vi "Readout.vi"(8 "Error In":errorcluster, 11 "BNT_DAQmx-MCSV in":refnum<class "BNT_DAQmx-MCSV.lvclass">) -> (0 "Error Out":errorcluster, 2 "CSPP_DataCollection out":refnum<class "CSPP_DataCollection.lvclass">, 3 "BNT_DAQmx-MCSV out":refnum<class "BNT_DAQmx-MCSV.lvclass">)   [LabVIEW 2019, in "BNT_DAQmx.lvlib" / "BNT_DAQmx-MCSV.lvclass"]
doc: "Read single value from multiple channels."
uses:
  BNT_DAQmx-MCSV.lvclass
  CSPP_Core/Classes/CSPP_BaseClasses/DataCollection/CSPP_DataCollection.lvclass
  C:/User/Brand/LVP/LaserSpec/RADRIS/Packages/CSPP_Core/Actors/CSPP_BaseActor/CSPP_BaseActor.lvclass
  C:/Program Files (x86)/National Instruments/LabVIEW 2019/vi.lib/ActorFramework/Actor/Actor.lvclass
  CSPP_Core/Messages/CSPP_DataUpdate Msg/CSPP_DataUpdate Msg.lvclass
  BNT_DAQmx-MCSV-Data/BNT_DAQmx-MCSV-Data.lvclass
  C:/User/Brand/LVP/LaserSpec/RADRIS/Packages/CSPP_Core/Classes/CSPP_BaseClasses/Data/CSPP_Data.lvclass
  BNT_DAQmx-MCSV.lvclass/BNT_DAQmx-MCSV.ctl
  CSPP_Core/Actors/CSPP_BaseActor/CSPP_BaseActor.lvclass/CSPP_BaseActor.ctl
  CSPP_Core/Classes/CSPP_BaseClasses/Data/CSPP_Data.lvclass/CSPP_Data.ctl
  CSPP_Core/Classes/CSPP_BaseClasses/DataCollection/CSPP_DataCollection.lvclass/CSPP_DataCollection.ctl
  <vilib>/ActorFramework/Actor/Actor.lvclass/Actor.ctl
  <vilib>/ActorFramework/Message Enqueuer/Message Enqueuer.lvclass/Message Enqueuer.ctl
  <vilib>/DAQmx/read.llb/DAQmx Read (Counter 1D DBL NChan 1Samp).vi
  <vilib>/DAQmx/read.llb/DAQmx Read (Digital 1D Bool 1Chan 1Samp).vi
  CSPP_Core/Classes/CSPP_BaseClasses/Data/Write Error.vi
  CSPP_Core/Classes/CSPP_BaseClasses/Data/Write Time Stamp.vi
  <vilib>/ActorFramework/Message Enqueuer/Init from Existing Queue.vi
  <vilib>/DAQmx/miscellaneous.llb/DAQmx Fill In Error Info.vi
  <vilib>/ActorFramework/Message Enqueuer/Message Enqueuer.lvclass
  CSPP_Core/Actors/CSPP_BaseActor/CSPP_BaseActor.lvclass
  <vilib>/ActorFramework/Actor/Actor.lvclass
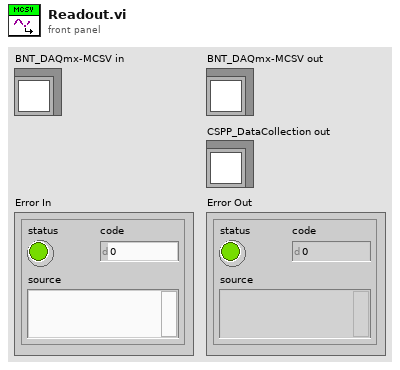
[diagram p1: front panel]
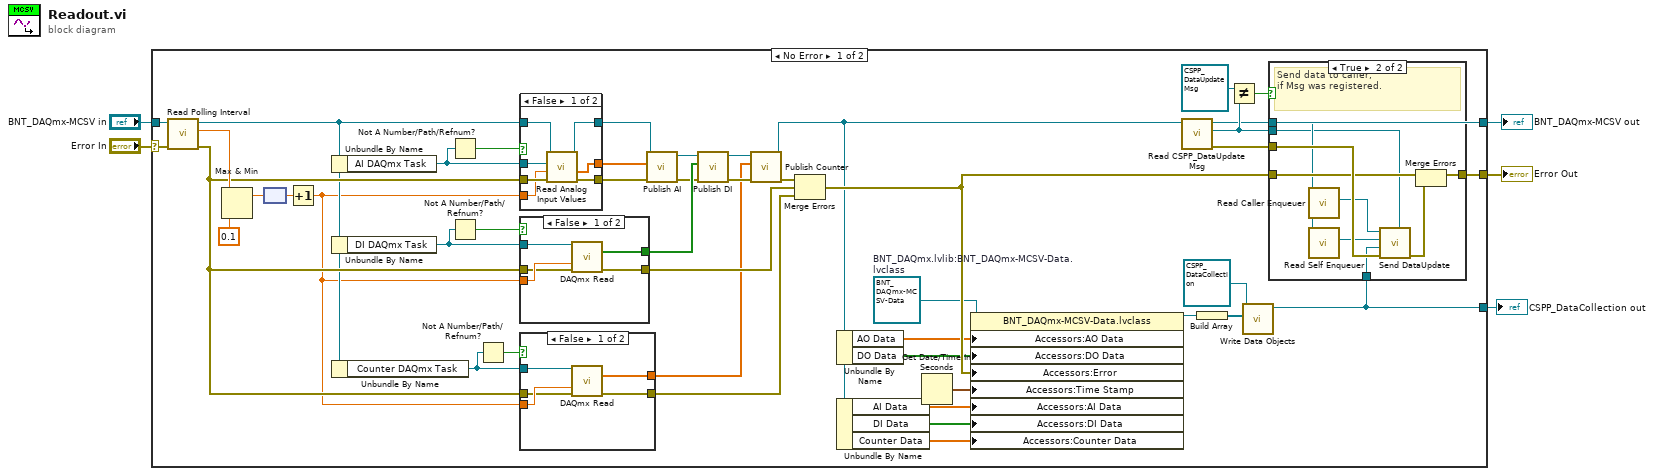
[diagram p0: block diagram]
diagram:
  n1 = case shown="No Error" "Error In" {
    selector: "Error In" -> [w50 w84]
    tunnel: [w38 w84] -> w4
    tunnel: [w20 w83] -> w2
    tunnel: "BNT_DAQmx-MCSV in" -> [w51 w83]
    tunnel: [w25 _] -> w1
    frame No Error {
      w32 = refnum<class "BNT_DAQmx-MCSV-Data.lvclass"> refnum  # BNT_DAQmx.lvlib:BNT_DAQmx-MCSV-Data.lvclass
      n2 = call "Read Polling Interval.vi"("error in (no error)"=w50, "CSPP_BaseActor in"=w51) -> ("error out"=w37:errorcluster, "Polling Interval"=w49:dbl[unit], "CSPP_BaseActor out"=w23:refnum<class "BNT_DAQmx-MCSV.lvclass">)  [unwired: 7 in]
      n3 = Max & Min(x=w49, y=dbl[unit] 0.1) -> (max(x,y)=w47:dbl[unit])  [unwired: 1 out]
      n4 = node(w47) -> (w40:dbl)
      n5 = Increment(x=w40) -> (x+1=w21:dbl)
      n6 = Unbundle By Name(w23) -> ("AI DAQmx Task"=w22:refnum<k21>)
      n7 = Unbundle By Name(w23) -> ("DI DAQmx Task"=w44:refnum<k21>)
      n8 = Unbundle By Name(w23) -> ("Counter DAQmx Task"=w41:refnum<k21>)
      n9 = Not A Number/Path/Refnum?(number/path/refnum=w22) -> (NaN/Path/Refnum?=w45:bool)
      n10 = Not A Number/Path/Refnum?(number/path/refnum=w44) -> (NaN/Path/Refnum?=w43:bool)
      n11 = Not A Number/Path/Refnum?(number/path/refnum=w41) -> (NaN/Path/Refnum?=w42:bool)
      n12 = case shown="False" w45 {
        tunnel: [w59 w66] -> w17
        tunnel: w21 -> [w62 _]
        tunnel: w37 -> [w63 w66]
        tunnel: w23 -> [w64 w65]
        tunnel: [w60 w65] -> w18
        tunnel: w22 -> [w61 _]
        tunnel: [w58 _] -> w16
        frame False {
          n13 = call-dynamic "Read Analog Input Values.vi"("error in"=w63, "Timeout / s"=w62, "AI DAQmx Task"=w61, "BNT_DAQmx-MCSV in"=w64) -> ("error out"=w59:errorcluster, "AI Data"=w58:dbl[], "BNT_DAQmx-MCSV out"=w60:refnum<class "BNT_DAQmx-MCSV.lvclass">)  [unwired: 5 in]
        }
        frame True {
        }
      }
      n14 = case shown="False" w43 {
        tunnel: w44 -> [w56 _]
        tunnel: w21 -> [w55 _]
        tunnel: [w52 _] -> w14
        tunnel: [w53 w57] -> w46
        tunnel: w37 -> [w54 w57]
        frame False {
          n15 = call-poly <vilib>:"DAQmx Read.vi"("task/channels in"=w56, "timeout"=w55, "error in"=w54) -> ("data"=w52:bool[], "error out"=w53:errorcluster)  [unwired: 10 in, 1 out]
        }
        frame True {
        }
      }
      n16 = case shown="False" w42 {
        tunnel: w41 -> [w71 _]
        tunnel: w21 -> [w70 _]
        tunnel: [w67 _] -> w8
        tunnel: [w68 w72] -> w39
        tunnel: w37 -> [w69 w72]
        frame False {
          n17 = call-poly <vilib>:"DAQmx Read.vi"("task/channels in"=w71, "timeout"=w70, "error in"=w69) -> ("data"=w67:dbl[], "error out"=w68:errorcluster)  [unwired: 10 in, 1 out]
        }
        frame True {
        }
      }
      n18 = call "Publish AI.vi"("error in"=w17, "AI Data"=w16, "BNT_DAQmx-MCSV in"=w18) -> ("error out"=w13:errorcluster, "BNT_DAQmx-MCSV out"=w12:refnum<class "BNT_DAQmx-MCSV.lvclass">)  [unwired: 7 in]
      n19 = call "Publish DI.vi"("error in"=w13, "DI Data"=w14, "BNT_DAQmx-MCSV in"=w12) -> ("error out"=w10:errorcluster, "BNT_DAQmx-MCSV out"=w11:refnum<class "BNT_DAQmx-MCSV.lvclass">)  [unwired: 7 in]
      n20 = call "Publish Counter.vi"("error in"=w10, "Counter Data"=w8, "BNT_DAQmx-MCSV in"=w11) -> ("error out"=w9:errorcluster, "BNT_DAQmx-MCSV out"=w6:refnum<class "BNT_DAQmx-MCSV.lvclass">)  [unwired: 7 in]
      n21 = Merge Errors(w9, w46, w39) -> (w35:errorcluster)
      n22 = Unbundle By Name(w6) -> ("AO Data"=w30:dbl[], "DO Data"=w29:bool[])
      n23 = Unbundle By Name(w6) -> ("AI Data"=w19:dbl[], "DI Data"=w15:bool[], "Counter Data"=w7:dbl[])
      n24 = Get Date/Time In Seconds() -> (seconds since 1Jan1904=w31:timestamp)
      n25 = property class="BNT_DAQmx-MCSV-Data.lvclass"(reference=w32, "Accessors:AO Data"=w30, "Accessors:DO Data"=w29, "Accessors:Error"=w35, "Accessors:Time Stamp"=w31, "Accessors:AI Data"=w19, "Accessors:DI Data"=w15, "Accessors:Counter Data"=w7) -> (reference out=w27:refnum<class "BNT_DAQmx-MCSV-Data.lvclass">)  [unwired: 1 in, 1 out]
      n26 = call-dynamic "Read CSPP_DataUpdate Msg.vi"("CSPP_BaseActor in"=w6) -> ("error out"=w36:errorcluster, "CSPP_DataUpdate Msg.lvclass"=w34:refnum<class "CSPP_DataUpdate Msg.lvclass">, "CSPP_BaseActor out"=w20:refnum<class "BNT_DAQmx-MCSV.lvclass">)  [unwired: 8 in]
      n27 = Build Array(w27) -> (w26:refnum<class "BNT_DAQmx-MCSV-Data.lvclass">[])
      n28 = Not Equal?(x=refnum<class "CSPP_DataUpdate Msg.lvclass"> refnum ("CSPP_DataUpdate Msg.lvclass"), y=w34) -> (x != y?=w24:bool)
      n29 = call "Write Data Objects.vi"("Data Objects"=w26, "CSPP_DataCollection in"=refnum<class "CSPP_DataCollection.lvclass"> refnum ("CSPP_BaseClasses.lvlib:CSPP_DataCollection.lvclass")) -> ("CSPP_DataCollection out"=w25:refnum<class "CSPP_DataCollection.lvclass">)  [unwired: 8 in, 1 out]
      n30 = case shown="True" w24 {
        tunnel: [w73 w82] -> w38
        tunnel: w36 -> [_ w81]
        tunnel: w35 -> [w73 w80]
        tunnel: w20 -> [_ w79]
        tunnel: w34 -> [_ w78]
        tunnel: w25 -> [_ w74]
        frame False {
        }
        frame True {
          # "Send data to caller, \nif Msg was registered."
          n31 = call <vilib>:"Read Caller Enqueuer.vi"("Actor"=w79) -> ("Caller Enqueuer"=w77:refnum<class "Message Enqueuer.lvclass">)  [unwired: 10 in]
          n32 = call <vilib>:"Read Self Enqueuer.vi"("Actor"=w79) -> ("Self Enqueuer"=w76:refnum<class "Message Enqueuer.lvclass">)  [unwired: 10 in]
          n33 = call "Send DataUpdate.vi"("CSPP_DataUpdate Msg"=w78, "error in (no error)"=w81, "CSPP_DataCollection"=w74, "Sender Enqueuer"=w76, "Message Enqueuer"=w77) -> ("error out"=w75:errorcluster)  [unwired: 5 in, 1 out]
          n34 = Merge Errors(w80, w75) -> (w82:errorcluster)
        }
      }
    }
    frame Error {
    }
  }
  "Error Out" <- w4
  "BNT_DAQmx-MCSV out" <- w2
  "CSPP_DataCollection out" <- w1
